vi "FGV_Polar_Array.vi"(8 "error in":errorcluster, 10 "Action":T1=enum."Read", 11 "Polar_Array IN":dbl[][](array[numeric])) -> (0 "error out":errorcluster, 2 "Polar size":i32=8, 3 "Polar_Array OUT":dbl[][](array[numeric])=[[0.0, 1.0, -1.0, 0.0, 0.5, -0.5], [1.0, -1.0, 0.0, 0.2, 0.8, 0.5], [-1.0, 0.0, 1.0, 0.3, 0.2, -0.5], [0.0, 1.0, 0.2, 0.4, -0.5, 0.5], [1.0, -0.5, 0.0, 0.5, -0.3, -0.5], [-0.5, 1.0, 0.0, -0.6, -1.0, 0.5], [0.0, 1.0, 0.9, -1.0, 1.0, -0.5], [1.0, 0.5, 0.0, 1.0, 0.7, 0.5]])   [LabVIEW 2026]
doc: "Functional Global Variable:\n- Write the value into the memory \nor\n- Read the value from the memory"
uses:
  TypeDef_FGV.ctl
panel:
  in  "Polar_Array Init":dbl[][](array[numeric])=[[0.0, 1.0, -1.0, 0.0, 0.5], [1.0, -1.0, 0.0, 0.2, 0.8], [-1.0, 0.0, 1.0, 0.3, 0.2], [0.0, 1.0, 0.2, 0.4, -0.5], [1.0, -0.5, 0.0, 0.5, -0.3], [-0.5, 1.0, 0.0, -0.6, -1.0], [0.0, 1.0, 0.9, -1.0, 1.0], [1.0, 0.5, 0.0, 1.0, 0.7]]
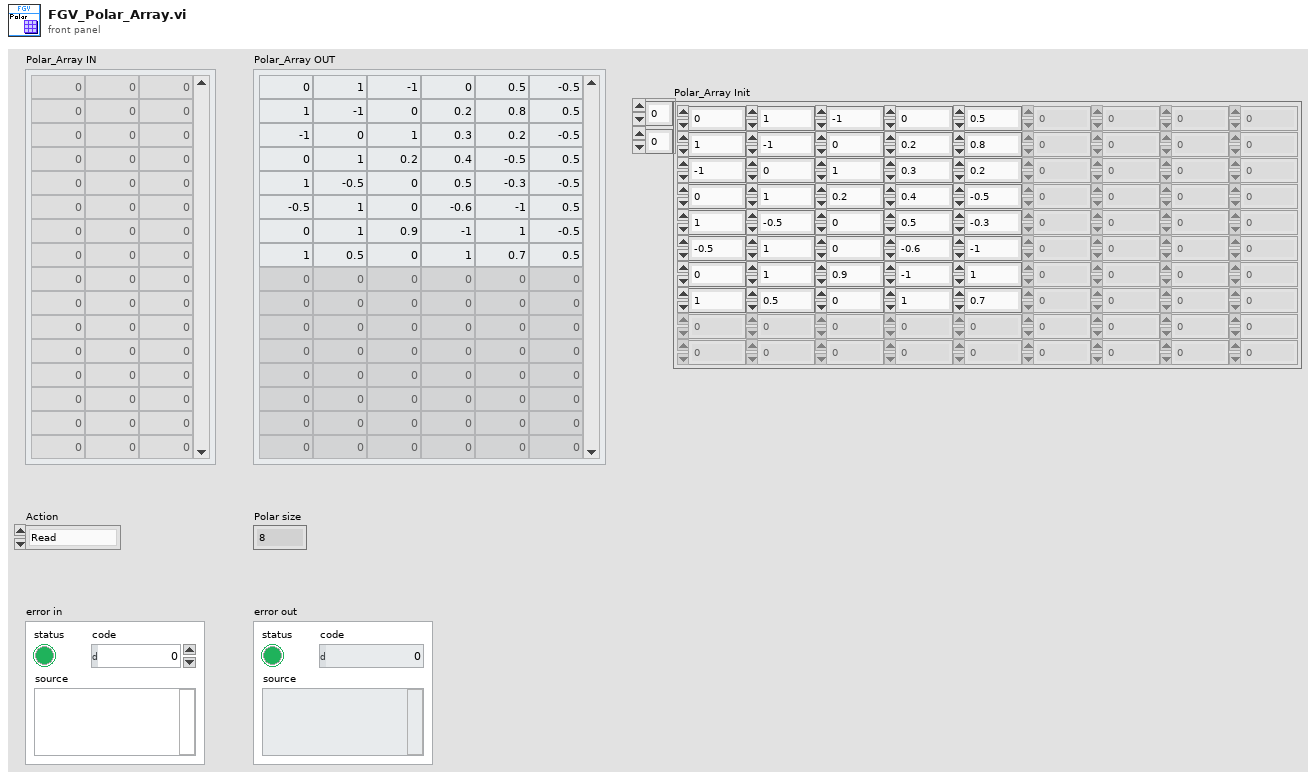
[diagram p1: front panel]
types:
  T1 = typedef "TypeDef_FGV.ctl" = enum16{"Initialize", "Write", "Read", "Read_File", "Write_to_File"}
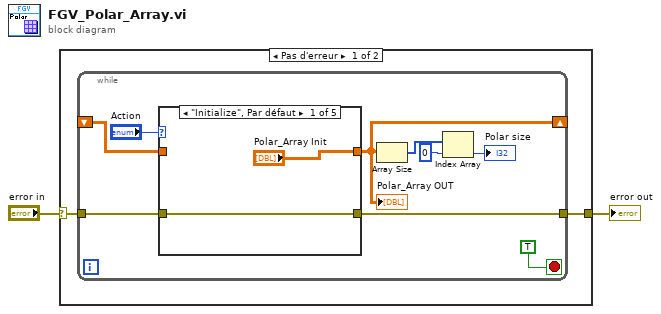
[diagram p0: block diagram]
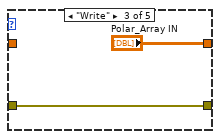
[diagram p3: hidden frame]
diagram:
  n1 = case shown="Pas d'erreur" "error in" {
    selector: "error in" -> [w4 w24]
    tunnel: [w3 w24] -> w1
    frame No Error {
      n2 = while {
        shift-right: [w10] -> _
        shift-left: _ -> [w11]
        tunnel: w4 -> [w6]
        tunnel: [w5] -> w3
        stop <- TRUE stop-if-true
        n3 = case shown="\"Initialize\", Par défaut" "Action" {
          tunnel: w11 -> [_ w17 _ w21 w23]
          tunnel: ["Polar_Array Init" w17 "Polar_Array IN" w21 w23] -> w10
          tunnel: w6 -> [w15 w16 w18 w20 w22]
          tunnel: [w15 w16 w18 w20 w22] -> w5
          frame "Initialize", Default {
          }
          frame "Read" {
          }
          frame "Write" {
          }
          frame "Read_File" {
            # "A FAIRE"
          }
          frame "Write_to_File" {
            # "A Faire"
          }
        }
        "Polar_Array OUT" <- w10
        n4 = Array Size(array=w10) -> (size(s)=w9:i32[])
        n5 = Index Array(array=w9, index=0) -> (element=→"Polar size":i32)
      }
    }
    frame Error {
    }
  }
  "error out" <- w1
